vi "Stop Event Handler.vi"(8 "error in (no error)":errorcluster, 11 "ActorAutoRegistration In":refnum<class "ActorAutoRegistration.lvclass">) -> (0 "error out":errorcluster)   [LabVIEW 2015, in "ActorAutoRegistration.lvlib" / "ActorAutoRegistration.lvclass"]
doc: "<License>\nCopyright © 2017 Composed Systems, LLC | All rights reserved\nwww.composed.io\n\nAuthor: Ethan Stern <ethan.stern@composed.io>\n\nThis software is provided \"AS IS\" WITHOUT WARRANTIES, either express or implied, AND IS FOR EDUCATIONAL PURPOSES ONLY.\n</License>"
uses:
  ActorAutoRegistration.lvclass
  ActorAutoRegistration.lvclass/ActorAutoRegistration.ctl
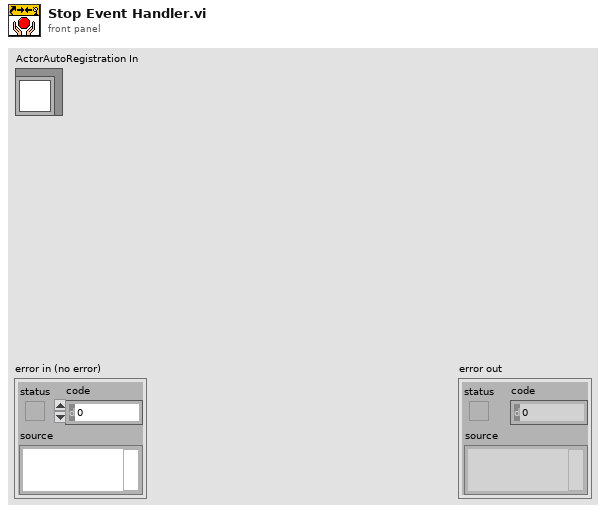
[diagram p1: front panel]
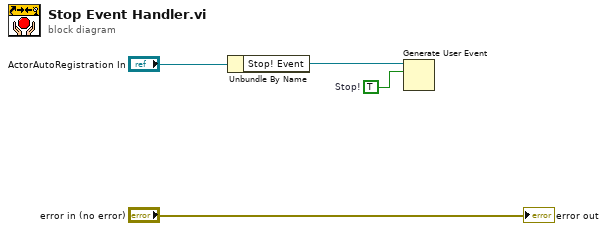
[diagram p0: block diagram]
diagram:
  w1 = TRUE  # Stop!
  n1 = Unbundle By Name("ActorAutoRegistration In") -> ("Stop! Event"=w2:refnum<user-event>)
  n2 = Generate User Event(user event=w2, event data cluster=w1) -> ()  [unwired: 2 in, 2 out]
  "error out" <- "error in (no error)"
